vi "view_3d_script.vi"(4 "center":cluster{"x":dbl, "y":dbl}, 5 "variables":dbl[](array[numeric]), 6 "script":string, 7 "vy in":T1(array[cluster]), 8 "picyure in":picture) -> (0 "boundaries":T2(array[cluster]), 2 "vy out":T1(array[cluster]), 3 "picture out":picture)   [LabVIEW 2011]
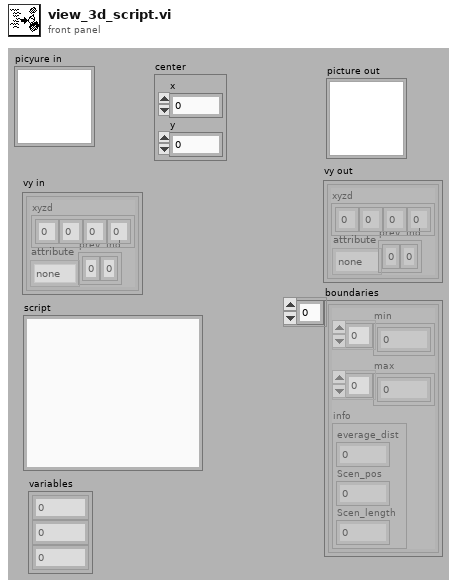
[diagram p1: front panel]
types:
  T1 = cluster{"xyzd":dbl[], "attribute":enum16{"none", "transparent", "reflective", "white", "black", "grey", "red", "yellow", "green", "blue", "pink"}, "prev. Ind.":i16[]}[]
  T2 = cluster{"min":dbl[], "max":dbl[], "info":cluster{"everage_dist":dbl, "Scen_pos":u16, "Scen_length":u16}}[]
  T3 = cluster{"xy_k_value":dbl[], "polygon":dbl[][], "attribute":enum16{"none", "transparent", "reflective", "white", "black", "grey", "red", "yellow", "green", "blue", "pink"}}[]
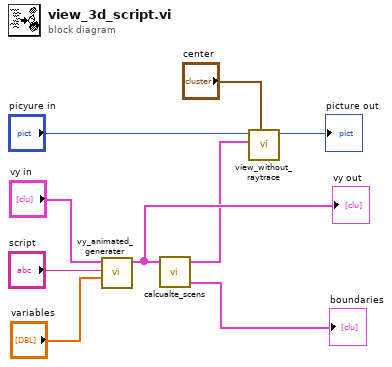
[diagram p0: block diagram]
diagram:
  n1 = call "vy_animated_generater.vi"("variables"="variables", "vy_string"="script", "vy_in"="vy in") -> ("vy_out"=w6:T1)  [unwired: 5 in, 1 out]
  "vy out" <- w6
  n2 = call "calcualte_scens.vi"("vy_in"=w6) -> ("boundaries"=→"boundaries":T2, "Scen out"=w2:T3)  [unwired: 3 in]
  n3 = call "view_without_raytrace.vi"("offset"="center", "Scens"=w2, "new picture"="picyure in") -> ("new picture 2"=→"picture out":picture)  [unwired: 6 in]
